vi "test_Create Data Channel_array existing channel name.vi"(8 "error in (no error)":errorcluster, 11 "TestCase in":refnum<class "Instrument Addon Scripting API Channels Unit Tests.lvclass">) -> (0 "error out":errorcluster, 3 "TestCase out":refnum<class "Instrument Addon Scripting API Channels Unit Tests.lvclass">)   [LabVIEW 2019, in "Instrument Addon Scripting API Channels Unit Tests.lvclass"]
uses:
  Instrument Addon Scripting API Channels Unit Tests.lvclass
  <vilib>/addons/_JKI Toolkits/VI Tester/TestCase.llb/TestCase.lvclass
  <vilib>/NI/NI VeriStand Advanced SysDef API/SysDef API/Advanced System Definition.lvlib
  Addon/Addon Shared/SubVIs/Constants.vi
  Addon/Addon Shared/Instrument Addon Shared.lvlib
  APIs/Scripting API/Instrument Addon Scripting API.lvlib
  APIs/Scripting API/TypeDefs/Array Element.ctl
  APIs/Scripting API/TypeDefs/Array Enumerated List Settings.ctl
  <vilib>/NI/NI VeriStand Advanced SysDef API/_SubVIs/SysDef.Search.GUID.vi
  APIs/Scripting API/Channels/Create Data Channel - Array - Enumerated List.vi
  <vilib>/NI/NI VeriStand Advanced SysDef API/_SubVIs/SysDef.Search.GUIDs.vi
  C:/Program Files (x86)/National Instruments/LabVIEW 2019/vi.lib/addons/_JKI Toolkits/VI Tester/TestCase.llb/TestCase.lvclass
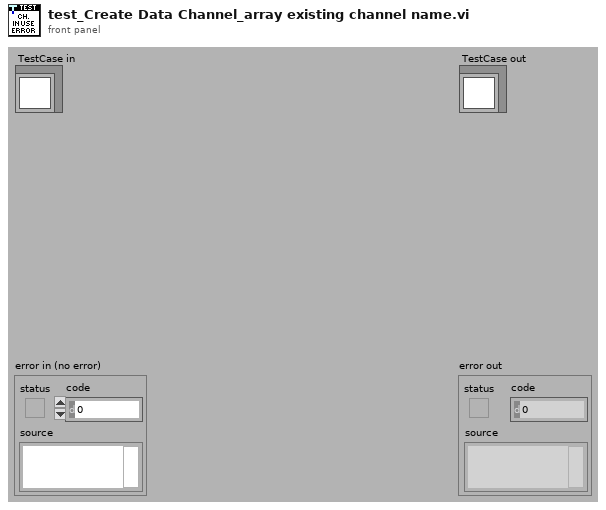
[diagram p1: front panel]
types:
  T1 = typedef "Instrument Addon Scripting API.lvlib/Array Enumerated List Settings.ctl" = cluster{"Elements":T2[], "Enumerated List":string[], "Delimiter":string}
  T2 = typedef "Instrument Addon Scripting API.lvlib/Array Element.ctl" = cluster{"Name":string, "Default Value":dbl, "Units":string}
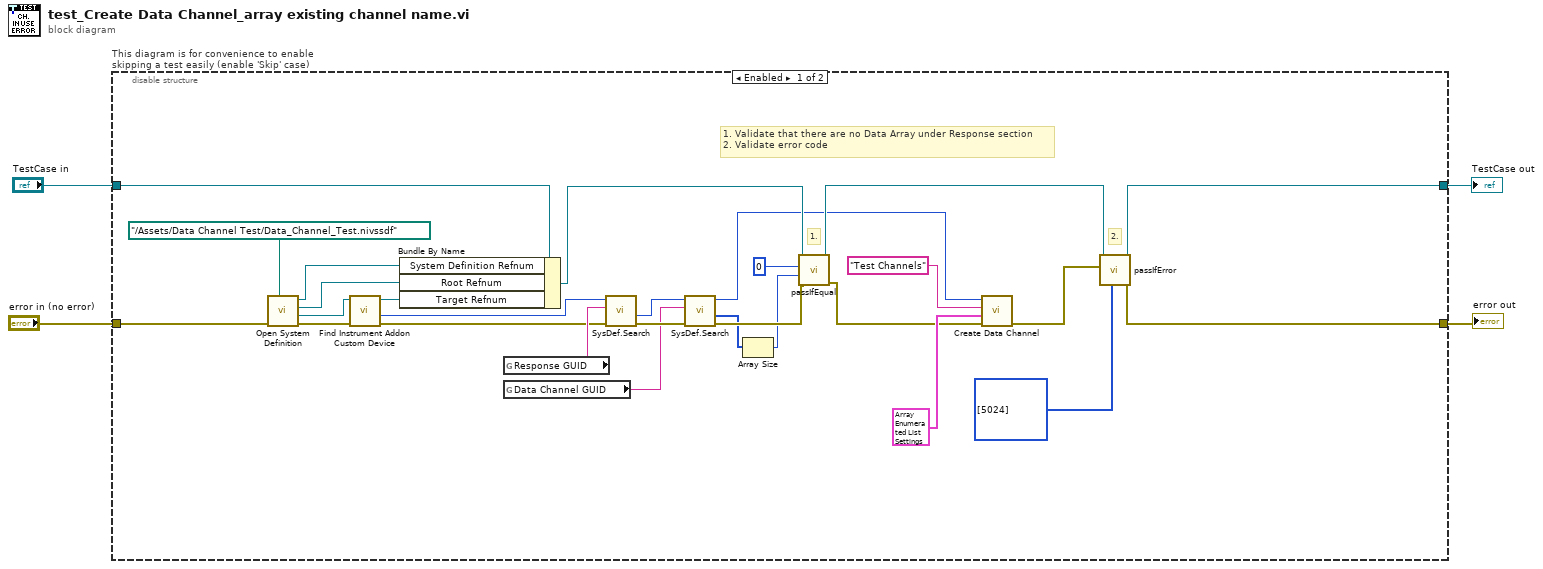
[diagram p0: block diagram]
diagram:
  n1 = disable-structure "This diagram is for convenience to enable skipping a test easily (enable 'Skip' case)" shown="Enabled" {
    disable-tunnel: "TestCase in" -> [w12 w36]
    disable-tunnel: [w14 w34] -> w1
    disable-tunnel: [w15 w35] -> w3
    disable-tunnel: "error in (no error)" -> [w29 w33]
    frame Enabled {
      # "2."
      # "1. Validate that there are no Data Array under Response section\n2. Validate error code"
      # "1."
      n2 = call "Open System Definition.vi"("error in (no error)"=w29, "System Definition File"=path "../Assets/Data Channel Test/Data_Channel_Test.nivssdf") -> ("error out"=w32:errorcluster, "Target Refnum"=w31:refnum<k24>, "Root Refnum"=w10:refnum<k24>, "System Definition Refnum"=w11:refnum<k24>)  [unwired: 6 in]
      n3 = call "Find Instrument Addon Custom Device.vi"("error in"=w32, "target in"=w31) -> ("error out"=w7:errorcluster, "NodeID"=w28:u64, "target out"=w9:refnum<k24>)  [unwired: 7 in]
      n4 = Bundle By Name(cluster=w12, "System Definition Refnum"=w11, "Root Refnum"=w10, "Target Refnum"=w9) -> (w8:refnum<class "Instrument Addon Scripting API Channels Unit Tests.lvclass">)
      n5 = global read "Constants.vi" "Response GUID"() -> (w27:string)
      n6 = global read "Constants.vi" "Data Channel GUID"() -> (w24:string)
      n7 = call-poly <vilib>:"SysDef.Search.vi"("error in (no error)"=w7, "GUID"=w27, "nodeID"=w28) -> ("error out"=w25:errorcluster, "Value out"=w26:u64)  [unwired: 5 in, 2 out]
      n8 = call-poly <vilib>:"SysDef.Search.vi"("error in (no error)"=w25, "GUID"=w24, "nodeID"=w26) -> ("error out"=w22:errorcluster, "Values Out"=w21:u64[], "nodeID out"=w5:u64)  [unwired: 5 in, 1 out]
      n9 = Array Size(array=w21) -> (size(s)=w20:i32)
      n10 = call-dynamic "passIfEqual.vi"("error in (no error)"=w22, "y"=w20, "x"=0 ("size(s)"), "TestCase in"=w8) -> ("error out"=w6:errorcluster, "TestCase out"=w23:refnum<class "Instrument Addon Scripting API Channels Unit Tests.lvclass">)  [unwired: 6 in]
      n11 = call-poly "Create Data Channel.vi"("error in (no error)"=w6, "settings"=T1 {"Elements"=[{"Name"="Scale", "Default Value"=10.0, "Units"="ms"}, {"Name"="Scale", "Default Value"=15.0, "Units"="ms"}], "Enumerated List"=["EnumListElement"], "Delimiter"="-"} ("Settings"), "channel name"="Test Channels" ("Name"), "response refnum in"=w5) -> ("error out"=w13:errorcluster)  [unwired: 4 in, 3 out]
      n12 = call-dynamic "passIfError.vi"("passing error codes (default = any error code)"=i32[] [5024], "error"=w13, "TestCase in"=w23) -> ("error out"=w15:errorcluster, "TestCase out"=w14:refnum<class "Instrument Addon Scripting API Channels Unit Tests.lvclass">)  [unwired: 7 in]
    }
    frame Disabled {
      # "skip test result while test is under development"
      n13 = call <vilib>:"skip.vi"("error in (no error)"=w33, "TestCase in"=w36) -> ("error out"=w35:errorcluster, "TestCase out"=w34:refnum<class "Instrument Addon Scripting API Channels Unit Tests.lvclass">)  [unwired: 8 in]
    }
  }
  "error out" <- w3
  "TestCase out" <- w1
